vi "GUIMessage.vi"() -> ()   [LabVIEW 2017]
uses:
  GUIMessage.ctl
panel:
  in  "GUIMessage":T1
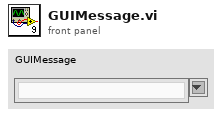
[diagram p1: front panel]
types:
  T1 = typedef "GUIMessage.ctl" = string
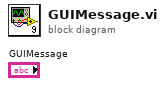
[diagram p0: block diagram]
diagram:
